vi "Cycle Params.vi"(6 "ID (Profile)":string="Profile", 7 "CYCLE params":T1={"ID"="", "Units"=enum."Metric", "RefPos"=0.0, "UpSpeed"=0.0, "DownSpeed"=0.0, "Distance"=0.0, "LoadStop"=0.0, "Direction"=enum."Up", "Autoreturn"=FALSE, "BreakStop"=FALSE, "HoldTimeEnd"=0.0, "HoldTimeRef"=0.0, "Mode"=enum."Time", "Time"=0.0, "Cycles"=1} {"Cycles" min=1 max=60000 step=1}, 8 "error in (no error)":errorcluster, 11 "Profile NO":u8=1 min=1 max=50 step=1) -> (0 "error out":errorcluster, 2 "wchitch params":string, 3 "params array out":string[](array[string]))   [LabVIEW 2019, in "STAV lib.lvlib"]
uses:
  STAV lib.lvlib
  Cycle params.ctl
  Param Units.ctl
  Param Direction.ctl
  Param Mode.ctl
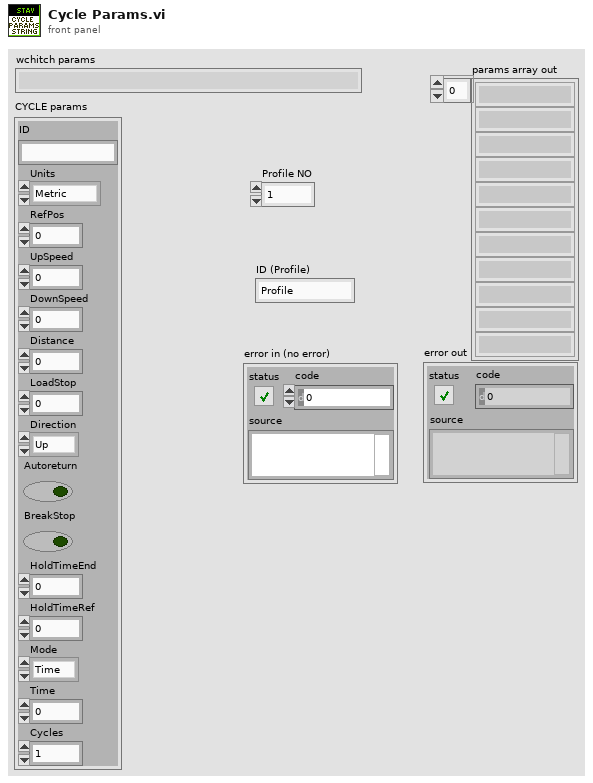
[diagram p1: front panel]
types:
  T1 = typedef "STAV lib.lvlib/Cycle params.ctl" = cluster{"ID":string, "Units":T2, "RefPos":dbl, "UpSpeed":dbl, "DownSpeed":dbl, "Distance":dbl, "LoadStop":dbl, "Direction":T3, "Autoreturn":bool, "BreakStop":bool, "HoldTimeEnd":dbl, "HoldTimeRef":dbl, "Mode":T4, "Time":dbl, "Cycles":i32}
  T2 = typedef "STAV lib.lvlib/Param Units.ctl" = enum16{"Metric", "Imperial"}
  T3 = typedef "STAV lib.lvlib/Param Direction.ctl" = enum16{"Up", "Down", "Left", "Right"}
  T4 = typedef "STAV lib.lvlib/Param Mode.ctl" = enum16{"Time", "Cycles"}
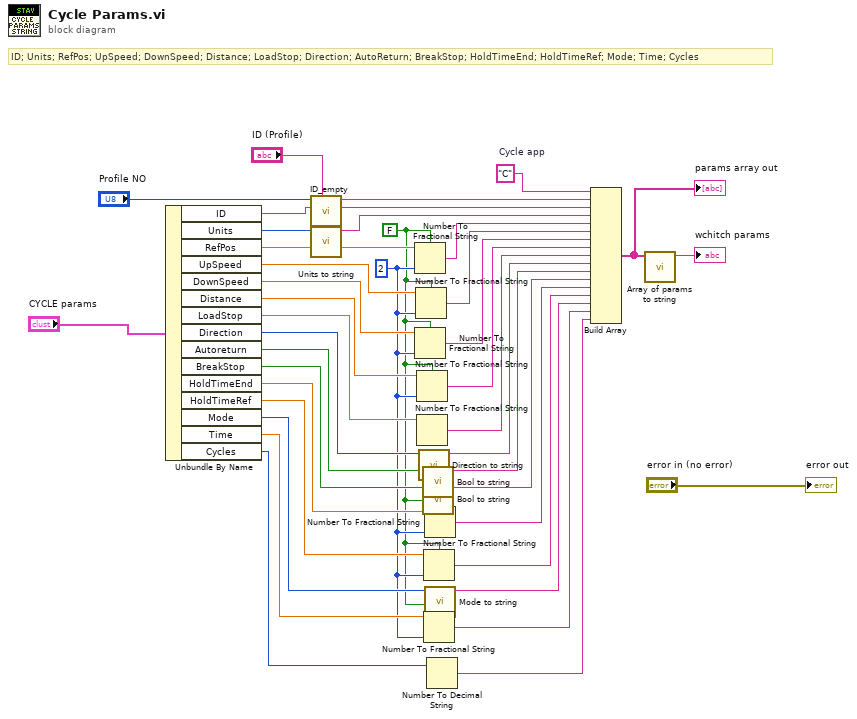
[diagram p0: block diagram]
diagram:
  w4 = i16 2 ("precision (6)")
  w3 = FALSE ("use system decimal point (T)")
  w40 = "C"  # Cycle app
  # "ID; Units; RefPos; UpSpeed; DownSpeed; Distance; LoadStop; Direction; AutoReturn; BreakStop; HoldTimeEnd; HoldTimeRef; Mode; Time; Cycles"
  n1 = Unbundle By Name("CYCLE params") -> ("ID"=w26:string, "Units"=w37:T2, "RefPos"=w36:dbl, "UpSpeed"=w33:dbl, "DownSpeed"=w32:dbl, "Distance"=w31:dbl, "LoadStop"=w20:dbl, "Direction"=w18:T3, "Autoreturn"=w16:bool, "BreakStop"=w14:bool, "HoldTimeEnd"=w12:dbl, "HoldTimeRef"=w11:dbl, "Mode"=w7:T4, "Time"=w10:dbl, "Cycles"=w2:i32)
  n2 = call "ID_empty.vi"("ID (Profile)"="ID (Profile)", "ID in"=w26, "Profile NO"="Profile NO") -> ("ID out"=w25:string, "Profile NO out"=w27:string)  [unwired: 7 in]
  n3 = call "Units to string.vi"("Units"=w37) -> ("Peak app"=w35:string)  [unwired: 10 in]
  n4 = Number To Fractional String(use system decimal point (T)=w3, number=w36, precision (6)=w4) -> (F-format string=w34:string)  [unwired: 1 in]
  n5 = Number To Fractional String(use system decimal point (T)=w3, number=w32, precision (6)=w4) -> (F-format string=w29:string)  [unwired: 1 in]
  n6 = Number To Fractional String(use system decimal point (T)=w3, number=w33, precision (6)=w4) -> (F-format string=w30:string)  [unwired: 1 in]
  n7 = Number To Fractional String(use system decimal point (T)=w3, number=w31, precision (6)=w4) -> (F-format string=w28:string)  [unwired: 1 in]
  n8 = Number To Fractional String(number=w20) -> (F-format string=w19:string)  [unwired: 3 in]
  n9 = call "Direction to string.vi"("Direction"=w18) -> ("Peak app"=w17:string)  [unwired: 10 in]
  n10 = call "Bool to string.vi"("Autoreturn"=w16) -> ("Peak app"=w15:string)  [unwired: 10 in]
  n11 = call "Bool to string.vi"("Autoreturn"=w14) -> ("Peak app"=w13:string)  [unwired: 10 in]
  n12 = Number To Fractional String(use system decimal point (T)=w3, number=w11, precision (6)=w4) -> (F-format string=w8:string)  [unwired: 1 in]
  n13 = Number To Fractional String(use system decimal point (T)=w3, number=w10, precision (6)=w4) -> (F-format string=w5:string)  [unwired: 1 in]
  n14 = Number To Fractional String(use system decimal point (T)=w3, number=w12, precision (6)=w4) -> (F-format string=w9:string)  [unwired: 1 in]
  n15 = call "Mode to string.vi"("Mode"=w7) -> ("String"=w6:string)  [unwired: 10 in]
  n16 = Number To Decimal String(number=w2) -> (decimal integer string=w1:string)  [unwired: 1 in]
  n17 = Build Array(w40, w27, w25, w35, w34, w30, w29, w28, w19, w17, w15, w13, w9, w8, w6, w5, w1) -> (w24:string[])
  "params array out" <- w24
  n18 = call "Array of params to string.vi"("Array"=w24) -> ("String"=→"wchitch params":string)  [unwired: 10 in]
  "error out" <- "error in (no error)"
